vi "getScanHardwareParameters.vi"(8 "error in (no error)":errorcluster, 11 "Microscope in":refnum<class "Microscope.lvclass">) -> (0 "error out":errorcluster, 2 "Scan Hardware Parameters":T1, 3 "Microscope out":refnum<class "Microscope.lvclass">)   [LabVIEW 2012, in "Microscope.lvclass"]
doc: "Gets hardware scan parameters such as image/s, s/image, clock rate and actual scan rate."
uses:
  classes/Microscope.lvclass
  classes/Microscope.lvclass/Microscope.ctl
  <resource>/objmgr/daqmx.rc
panel:
  in  "Cluster template":T1
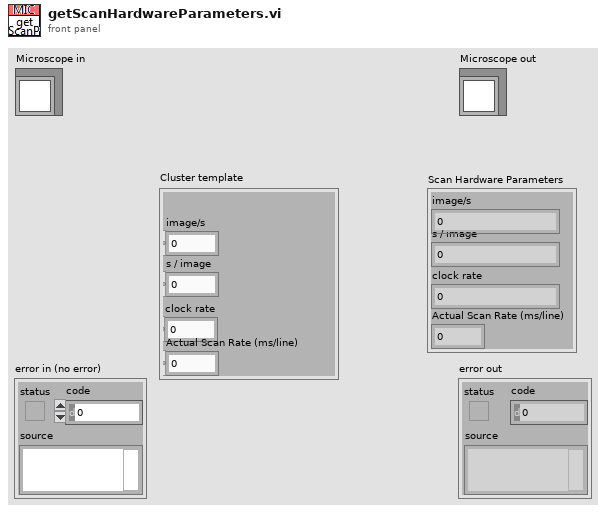
[diagram p1: front panel]
types:
  T1 = cluster{"s / image":dbl, "clock rate":dbl, "image/s":dbl, "Actual Scan Rate (ms/line)":dbl}
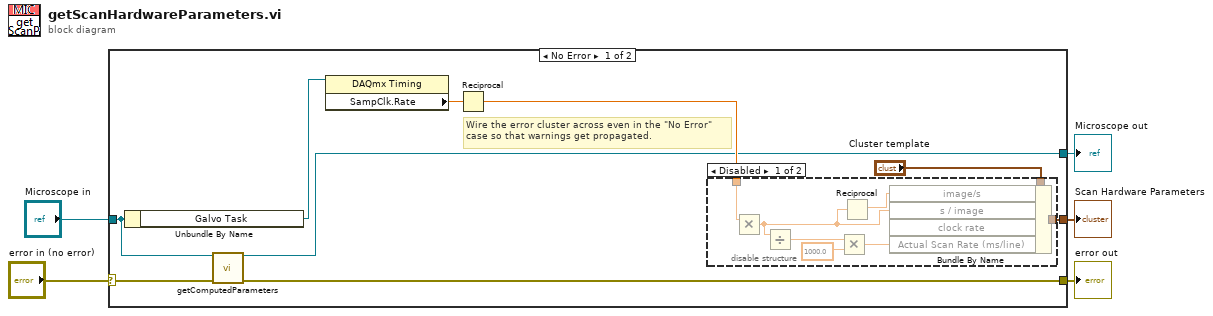
[diagram p0: block diagram]
diagram:
  n1 = case shown="No Error" "error in (no error)" {
    selector: "error in (no error)" -> [w9 w24]
    tunnel: [w8 w24] -> w4
    tunnel: [w10 w23] -> w2
    tunnel: "Microscope in" -> [w11 w23]
    tunnel: [w6 _] -> w1
    frame No Error {
      # "Wire the error cluster across even in the \"No Error\"\ncase so that warnings get propagated."
      n2 = Unbundle By Name(w11) -> ("Galvo Task"=w14:refnum<k21>)
      n3 = call "getComputedParameters.vi"("Microscope in"=w11, "error in (no error)"=w9) -> ("Microscope out"=w10:refnum<class "Microscope.lvclass">, "error out"=w8:errorcluster)  [unwired: 10 in, 2 out]
      n4 = property class="DAQmx Timing"(reference=w14) -> ("SampClk.Rate"=w13:dbl)  [unwired: 1 in, 2 out]
      n5 = Reciprocal(x=w13) -> (1/x=w12:dbl)
      n6 = disable-structure shown="Disabled" {
        disable-tunnel: w12 -> [w22 _]
        disable-tunnel: "Cluster template" -> [w21 _]
        disable-tunnel: [w20 _] -> w6
        frame Disabled {
          n7 = Multiply(x=w22) -> (x*y=w18:dbl)  [unwired: 1 in]
          n8 = Divide(x=w18) -> (x/y=w17:dbl)  [unwired: 1 in]
          n9 = Multiply(x=w17, y=1000.0) -> (x*y=w15:dbl)
          n10 = Reciprocal(x=w18) -> (1/x=w19:dbl)
          n11 = Bundle By Name(cluster=w21, "image/s"=w19, "s / image"=w18, "Actual Scan Rate (ms/line)"=w15) -> (w20:T1)  [unwired: 1 in]
        }
        frame Enabled {
        }
      }
    }
    frame Error {
    }
  }
  "error out" <- w4
  "Microscope out" <- w2
  "Scan Hardware Parameters" <- w1
